vi "ReadQualisysData.vi"(4 "sortie d'erreur":errorcluster caption="entrée d'erreur", 6 "QualisysDataType":enum16{"6DOF", "3DTracking", "6DOF + 3D"}(ring), 7 "QualisysFile":path) -> (0 "error out":errorcluster, 3 "Waveform Graph":waveform(dbl)[](graph))   [LabVIEW 2017]
panel:
  out "QualisysWaveforms":waveform(dbl)[](array[waveform])
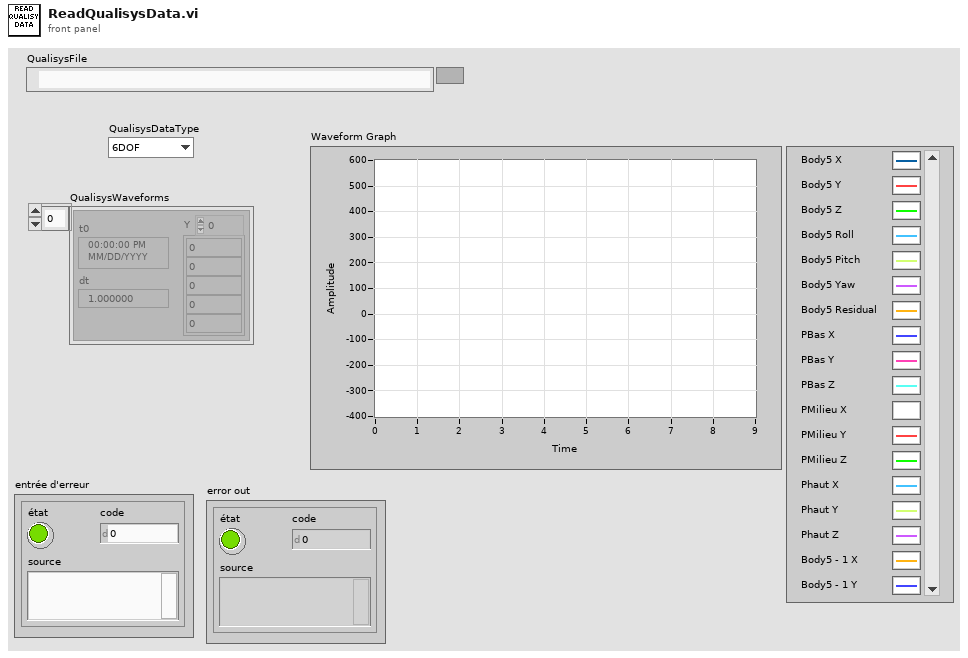
[diagram p1: front panel]
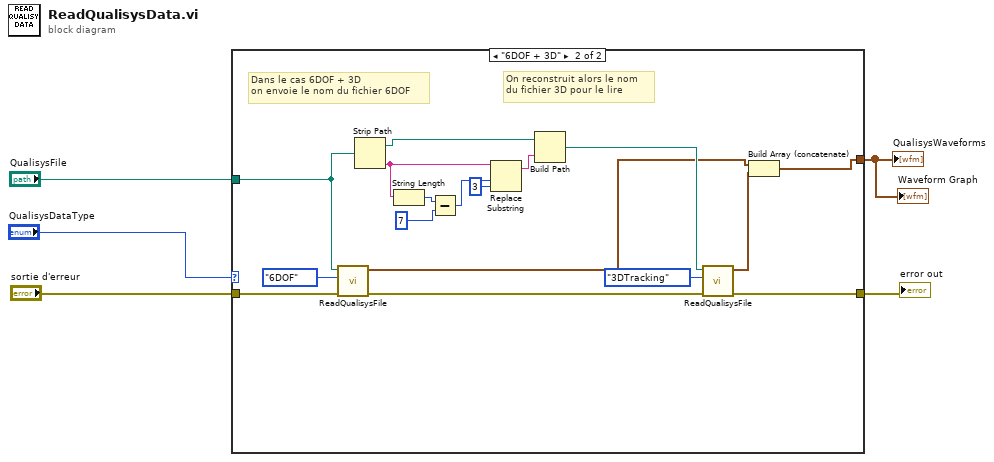
[diagram p0: block diagram]
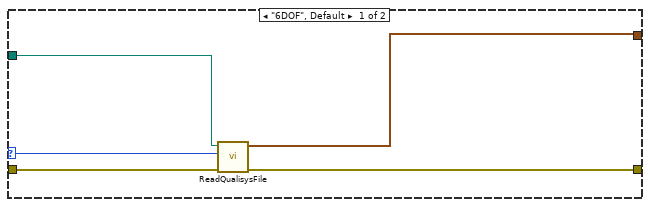
[diagram p2: hidden frame]
diagram:
  n1 = case shown="\"6DOF + 3D\"" "QualisysDataType" {
    selector: "QualisysDataType" -> [w7 _]
    tunnel: "QualisysFile" -> [w8 w25]
    tunnel: "sortie d'erreur" -> [w10 w27]
    tunnel: [w9 w16] -> w2
    tunnel: [w6 w11] -> w1
    frame "6DOF", Default {
      n2 = call "ReadQualisysFile.vi"("sortie d'erreur"=w10, "QualisysDataType"=w7, "FichierQualisys"=w8) -> ("error out"=w9:errorcluster, "QualisysWaveforms"=w6:waveform(dbl)[])  [unwired: 3 in]
    }
    frame "6DOF + 3D" {
      # "On reconstruit alors le nom \ndu fichier 3D pour le lire"
      # "Dans le cas 6DOF + 3D \non envoie le nom du fichier 6DOF"
      n3 = call "ReadQualisysFile.vi"("sortie d'erreur"=w27, "QualisysDataType"=enum16{"6DOF", "3DTracking", "6DOF + 3D"}."6DOF" ("QualisysDataType 2"), "FichierQualisys"=w25) -> ("error out"=w15:errorcluster, "QualisysWaveforms"=w13:waveform(dbl)[])  [unwired: 3 in]
      n4 = Strip Path(path=w25) -> (stripped path=w24:path, name=w23:string)
      n5 = String Length(string=w23) -> (length=w22:i32)
      n6 = Subtract(x=w22, y=7) -> (x-y=w20:i32)
      n7 = Replace Substring(2:3 ("length (len. of substring)"), 3:w20, 5:w23) -> (1:w18:string)  [unwired: 1 in, 1 out]
      n8 = Build Path(base path=w24, name or relative path=w18) -> (appended path=w14:path)
      n9 = call "ReadQualisysFile.vi"("sortie d'erreur"=w15, "QualisysDataType"=enum16{"6DOF", "3DTracking", "6DOF + 3D"}."3DTracking" ("QualisysDataType 2"), "FichierQualisys"=w14) -> ("error out"=w16:errorcluster, "QualisysWaveforms"=w12:waveform(dbl)[])  [unwired: 3 in]
      n10 = Build Array (concatenate)(w13, w12) -> (w11:waveform(dbl)[])
    }
  }
  "error out" <- w2
  "QualisysWaveforms" <- w1
  "Waveform Graph" <- w1
